vi "CMD_PICKPART.vi"(6 "Gantry in":refnum<class "Gantry.lvclass">, 8 "error in (no error)":errorcluster, 10 "Arguments":string[](array[string]), 11 "gScript Interpreter in":refnum<class "gScript Interpreter.lvclass">) -> (0 "error out":errorcluster, 3 "gScript Interpreter out":refnum<class "gScript Interpreter.lvclass">, 4 "Gantry out":refnum<class "Gantry.lvclass">)   [LabVIEW 2024, in "gScript Interpreter.lvclass"]
uses:
  gScript Interpreter.lvclass
  Shared Components/Gantry Class/Gantry.lvclass
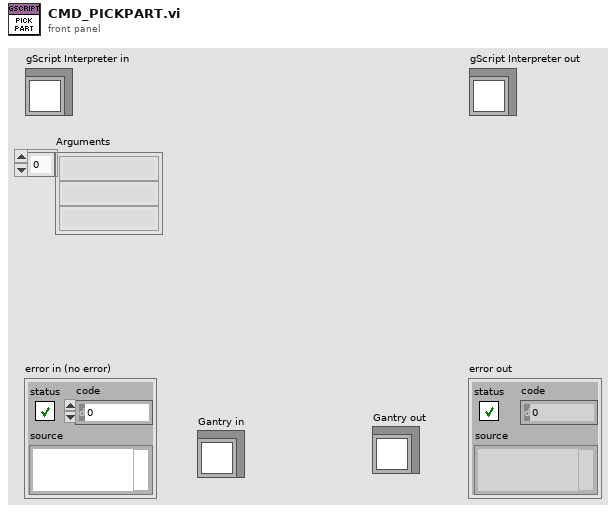
[diagram p1: front panel]
types:
  T1 = typedef "Memory Cell.ctl" = cluster{"type":T2, "x":dbl, "y":dbl, "z":dbl, "w":dbl}
  T2 = typedef "Memory Cell Type Enum.ctl" = enum16{"integer", "float", "vector", "rotation"}
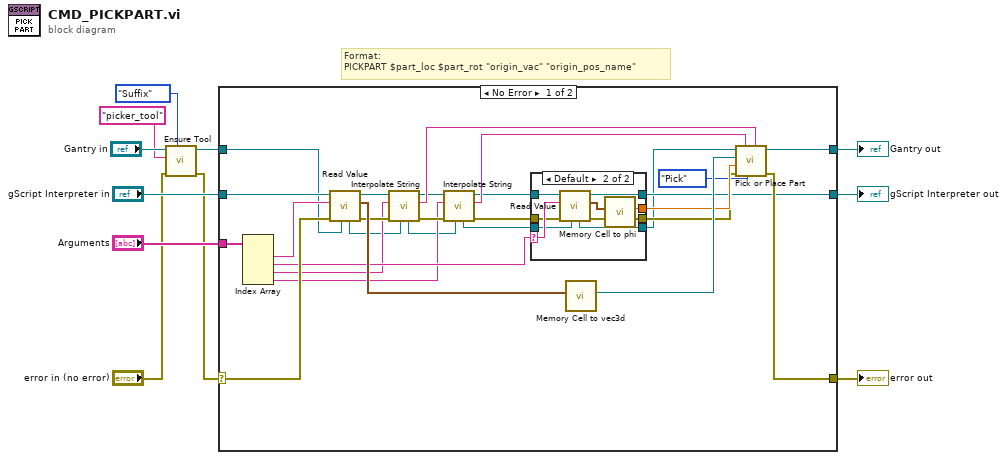
[diagram p0: block diagram]
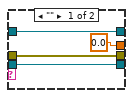
[diagram p2: hidden frame]
diagram:
  # "Format:\nPICKPART $part_loc $part_rot \"origin_vac\" \"origin_pos_name\""
  n1 = call "Ensure Tool.vi"("Match Type"=enum16{"Full", "Suffix"}."Suffix", "error in (no error)"="error in (no error)", "Tool Name"="picker_tool", "Gantry in"="Gantry in") -> ("error out"=w3:errorcluster, "Gantry out"=w5:refnum<class "Gantry.lvclass">)  [unwired: 6 in]
  n2 = case shown="No Error" w3 {
    selector: w3 -> [w36 w55]
    tunnel: [w28 w55] -> w11
    tunnel: [w27 w54] -> w9
    tunnel: "gScript Interpreter in" -> [w38 w54]
    tunnel: "Arguments" -> [w37 _]
    tunnel: w5 -> [w16 w53]
    tunnel: [w29 w53] -> w7
    frame No Error {
      n3 = Index Array(array=w37) -> (element #1=w39:string, element #2=w34:string, element #3=w24:string, element #4=w20:string)  [unwired: 4 in]
      n4 = call-dynamic "Read Value.vi"("Gantry in"=w16, "error in (no error)"=w36, "String in"=w39, "gScript Interpreter in"=w38) -> ("error out"=w25:errorcluster, "Memory Cell"=w35:T1, "gScript Interpreter out"=w26:refnum<class "gScript Interpreter.lvclass">, "Gantry out"=w15:refnum<class "Gantry.lvclass">)  [unwired: 4 in]
      n5 = call-dynamic "Interpolate String.vi"("Gantry in"=w15, "error in (no error)"=w25, "Input String"=w24, "gScript Interpreter in"=w26) -> ("error out"=w21:errorcluster, "Output String"=w23:string, "gScript Interpreter out"=w22:refnum<class "gScript Interpreter.lvclass">, "Gantry out"=w14:refnum<class "Gantry.lvclass">)  [unwired: 4 in]
      n6 = call-dynamic "Interpolate String.vi"("Gantry in"=w14, "error in (no error)"=w21, "Input String"=w20, "gScript Interpreter in"=w22) -> ("error out"=w18:errorcluster, "Output String"=w19:string, "gScript Interpreter out"=w17:refnum<class "gScript Interpreter.lvclass">, "Gantry out"=w13:refnum<class "Gantry.lvclass">)  [unwired: 4 in]
      n7 = case shown="Default" w34 {
        selector: w34 -> [_ w50]
        tunnel: w17 -> [w43 w52]
        tunnel: [w41 w51] -> w30
        tunnel: [0.0 ("float out") w48] -> w32
        tunnel: [w43 w47] -> w27
        tunnel: w18 -> [w41 w46]
        tunnel: w13 -> [w40 w45]
        tunnel: [w40 w44] -> w12
        frame "" {
        }
        frame Default {
          n8 = call-dynamic "Read Value.vi"("Gantry in"=w45, "error in (no error)"=w46, "String in"=w50, "gScript Interpreter in"=w52) -> ("error out"=w51:errorcluster, "Memory Cell"=w49:T1, "gScript Interpreter out"=w47:refnum<class "gScript Interpreter.lvclass">, "Gantry out"=w44:refnum<class "Gantry.lvclass">)  [unwired: 4 in]
          n9 = call "Memory Cell to phi.vi"("Memory Cell"=w49) -> ("float out"=w48:dbl)  [unwired: 10 in]
        }
      }
      n10 = call "Memory Cell to vec3d.vi"("Memory Cell"=w35) -> ("Vec3d out"=w33:refnum<class "Vec3d.lvclass">)  [unwired: 10 in]
      n11 = call "Pick or Place Part.vi"("Part Vacuum Line"=w23, "Pick or Place"=enum16{"Pick", "Place"}."Pick", "Part Named Position"=w19, "error in (no error)"=w30, "Part Rotation"=w32, "Part Position"=w33, "Gantry in"=w12) -> ("error out"=w28:errorcluster, "Gantry out"=w29:refnum<class "Gantry.lvclass">)  [unwired: 3 in]
    }
    frame Error {
    }
  }
  "error out" <- w11
  "gScript Interpreter out" <- w9
  "Gantry out" <- w7
